vi "findleftmostbitI16iter.vi"(1 "x":i16 format="%b") -> (0 "index":i16)   [LabVIEW 2018, in "posit.lvlib"]
uses:
  posit.lvlib
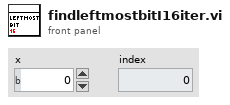
[diagram p1: front panel]
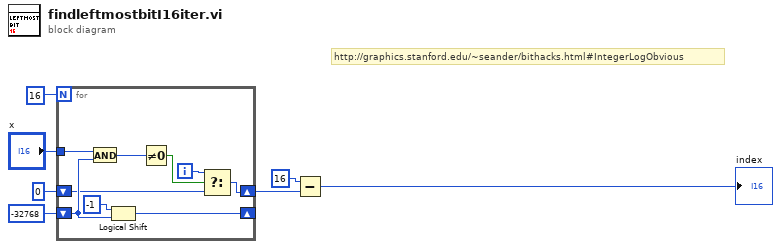
[diagram p0: block diagram]
diagram:
  # "http://graphics.stanford.edu/~seander/bithacks.html#IntegerLogObvious"
  n1 = for {
    N: 16 -> [_]
    tunnel: "x" -> [w16]
    shift-right: [w14] -> _
    shift-left: i16 -32768 -> [w12]
    shift-right: [w9] -> w2
    shift-left: 0 -> [w8]
    i -> [w10]
    n2 = And(x=w16, y=w12) -> (x .and. y?=w15:i16)
    n3 = Logical Shift(y=i16 -1, x=w12) -> (x << y=w14:i16)
    n4 = Not Equal To 0?(x=w15) -> (x != 0?=w11:bool)
    n5 = Select(t=w10, s=w11, f=w8) -> (s? t:f=w9:i32)
  }
  n6 = Subtract(x=16, y=w2) -> (x-y=→"index":i32)
